vi "find steer angle errors.vi"(10 "Desired Motion":T1, 11 "Actual Angles":T1) -> (3 "Commanded Motion":T1)   [LabVIEW 2018]
uses:
  Controls/Robot Pivot Motion Commands.ctl
  Controls/Pivot Motor Commands.ctl
  Controls/Robot Drive Mode.ctl
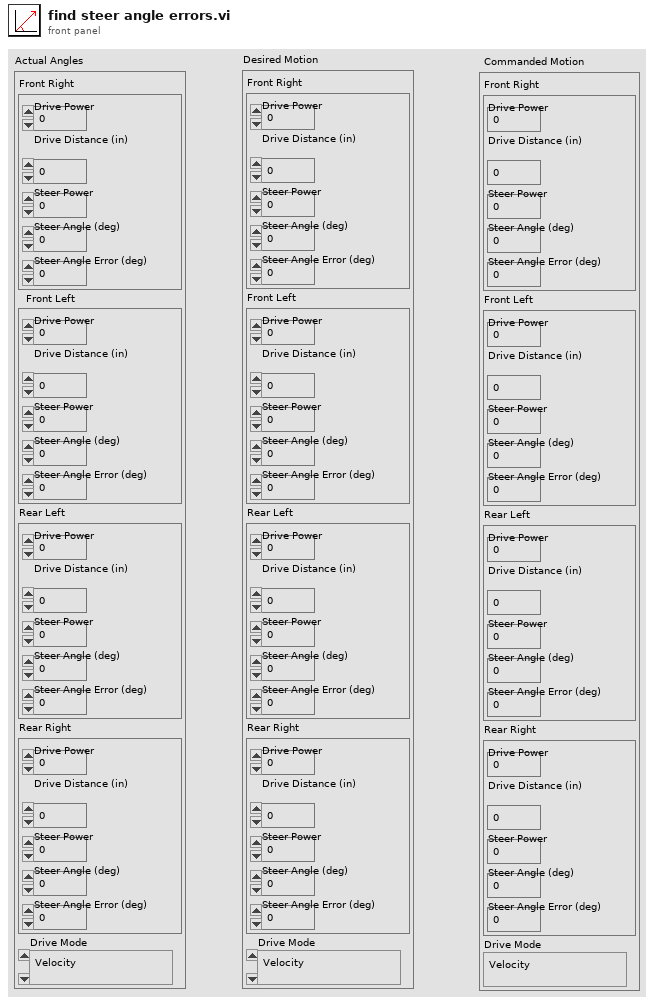
[diagram p1: front panel]
types:
  T1 = typedef "Robot Pivot Motion Commands.ctl" = cluster{"Front Right":T2, "Front Left":T2, "Rear Left":T2, "Rear Right":T2, "Drive Mode":T3}
  T2 = typedef "Pivot Motor Commands.ctl" = cluster{"Drive Power":dbl, "Drive Distance (in)":dbl, "Steer Power":dbl, "Steer Angle (deg)":dbl, "Steer Angle Error (deg)":dbl}
  T3 = typedef "Robot Drive Mode.ctl" = enum16{"Velocity", "Distance"}
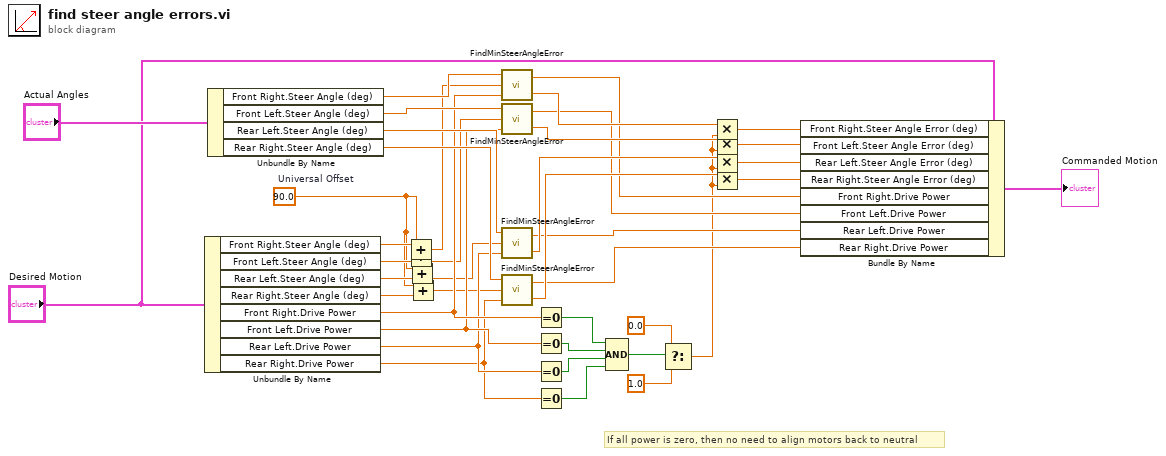
[diagram p0: block diagram]
diagram:
  w1 = 90.0  # Universal Offset
  # "If all power is zero, then no need to align motors back to neutral"
  n1 = Unbundle By Name("Desired Motion") -> ("Front Right.Steer Angle (deg)"=w35:dbl, "Front Left.Steer Angle (deg)"=w34:dbl, "Rear Left.Steer Angle (deg)"=w33:dbl, "Rear Right.Steer Angle (deg)"=w32:dbl, "Front Right.Drive Power"=w17:dbl, "Front Left.Drive Power"=w16:dbl, "Rear Left.Drive Power"=w15:dbl, "Rear Right.Drive Power"=w14:dbl)
  n2 = Unbundle By Name("Actual Angles") -> ("Front Right.Steer Angle (deg)"=w39:dbl, "Front Left.Steer Angle (deg)"=w38:dbl, "Rear Left.Steer Angle (deg)"=w37:dbl, "Rear Right.Steer Angle (deg)"=w36:dbl)
  n3 = Add(x=w35, y=w1) -> (x+y=w5:dbl)
  n4 = Add(x=w1, y=w34) -> (x+y=w4:dbl)
  n5 = Add(x=w1, y=w33) -> (x+y=w3:dbl)
  n6 = Add(x=w1, y=w32) -> (x+y=w2:dbl)
  n7 = call "FindMinSteerAngleError.vi"("Motor Power"=w17, "Desired Angle"=w5, "Actual Angle"=w39) -> ("Angle Error"=w29:dbl, "Motor Power"=w25:dbl)
  n8 = call "FindMinSteerAngleError.vi"("Motor Power"=w16, "Desired Angle"=w4, "Actual Angle"=w38) -> ("Angle Error"=w28:dbl, "Motor Power"=w24:dbl)
  n9 = call "FindMinSteerAngleError.vi"("Motor Power"=w15, "Desired Angle"=w3, "Actual Angle"=w37) -> ("Angle Error"=w27:dbl, "Motor Power"=w23:dbl)
  n10 = call "FindMinSteerAngleError.vi"("Motor Power"=w14, "Desired Angle"=w2, "Actual Angle"=w36) -> ("Angle Error"=w26:dbl, "Motor Power"=w22:dbl)
  n11 = Equal To 0?(x=w17) -> (x = 0?=w13:bool)
  n12 = Equal To 0?(x=w16) -> (x = 0?=w12:bool)
  n13 = Equal To 0?(x=w15) -> (x = 0?=w11:bool)
  n14 = Equal To 0?(x=w14) -> (x = 0?=w10:bool)
  n15 = Compound Arithmetic op=AND(w13, w12, w11, w10) -> (w9:bool)
  n16 = Select(t=0.0, s=w9, f=1.0) -> (s? t:f=w6:dbl)
  n17 = Multiply(x=w29, y=w6) -> (x*y=w21:dbl)
  n18 = Multiply(x=w28, y=w6) -> (x*y=w20:dbl)
  n19 = Multiply(x=w27, y=w6) -> (x*y=w19:dbl)
  n20 = Multiply(x=w26, y=w6) -> (x*y=w18:dbl)
  n21 = Bundle By Name(cluster="Desired Motion", "Front Right.Steer Angle Error (deg)"=w21, "Front Left.Steer Angle Error (deg)"=w20, "Rear Left.Steer Angle Error (deg)"=w19, "Rear Right.Steer Angle Error (deg)"=w18, "Front Right.Drive Power"=w25, "Front Left.Drive Power"=w24, "Rear Left.Drive Power"=w23, "Rear Right.Drive Power"=w22) -> (→"Commanded Motion":T1)
